vi "MouseDown.vi"(7 "Flip colors?":bool, 8 "error in":errorcluster, 10 "Coords":T5, 11 "Data in":T1={"Class"={"Ants"=refnum, "Layer"=refnum, "Templates"=refnum, "Icon"=refnum, "Glyph"=refnum, "Settings"=refnum, "Tools"=refnum, "History"=refnum}, "Ref"={"Add Layer"=refnum, "Remove Layer"=refnum, "Line Text"=[], "Body Text Spec"=refnum, "DNL_Font"=refnum, "glyph path str"=refnum, "templates path str"=refnum, "Arrow Up"=refnum, "Arrow Down"=refnum, "IE VI Ref"=refnum, "Glyphs tree"=refnum, "Templates tree"=refnum, "Layer Icon Text"=refnum, "Layer Template"=refnum, "Body Text"=refnum, "Search Templates"=refnum, "TextMarker"=refnum, "Tab Control"=refnum, "Search Glyphs"=refnum, "Line Color"=refnum, "DNL_Glyphs []"=refnum, "Fill Color"=refnum, "Tools"=refnum, "Icon"=refnum, "Preview"=refnum, "Ants"=refnum, "Terminals"=refnum, "menu reference"=refnum, "LayerNames"=[], "GlyphLoadAnimation"=refnum, "TemplateLoadAnimation"=refnum, "refreshGlyphs"=refnum, "refreshTemplates"=refnum}, "Support"={"AntsRect"={"left"=0, "top"=0, "right"=0, "bottom"=0}, "Mouse Move Coords"={"Horizontal"=0, "Vertical"=0}, "Mouse Down Coords"={"Horizontal"=0, "Vertical"=0}, "Temp Coord"={"Horizontal"=0, "Vertical"=0}, "Action"=enum."Default", "Edge Color"=4914962, "Fill Color"=16860, "Mouse Down?"=FALSE, "Draft Mode?"=FALSE, "Temp Icon"=bytes[3102], "CTRL Pressed"=FALSE, "Move Selection?"=FALSE, "AntsRect Orig"={"left"=0, "top"=0, "right"=0, "bottom"=0}, "Text"="", "TM Set?"=FALSE, "Mouse inside icon?"=FALSE, "Tool (old value)"=0, "Pencil Move Color"=0, "Swap Colors?"=FALSE, "Shift pressed?"=FALSE}}) -> (0 "error out":errorcluster, 3 "Data out":T1={"Class"={"Ants"=refnum, "Layer"=refnum, "Templates"=refnum, "Icon"=refnum, "Glyph"=refnum, "Settings"=refnum, "Tools"=refnum, "History"=refnum}, "Ref"={"Add Layer"=refnum, "Remove Layer"=refnum, "Line Text"=[], "Body Text Spec"=refnum, "DNL_Font"=refnum, "glyph path str"=refnum, "templates path str"=refnum, "Arrow Up"=refnum, "Arrow Down"=refnum, "IE VI Ref"=refnum, "Glyphs tree"=refnum, "Templates tree"=refnum, "Layer Icon Text"=refnum, "Layer Template"=refnum, "Body Text"=refnum, "Search Templates"=refnum, "TextMarker"=refnum, "Tab Control"=refnum, "Search Glyphs"=refnum, "Line Color"=refnum, "DNL_Glyphs []"=refnum, "Fill Color"=refnum, "Tools"=refnum, "Icon"=refnum, "Preview"=refnum, "Ants"=refnum, "Terminals"=refnum, "menu reference"=refnum, "LayerNames"=[], "GlyphLoadAnimation"=refnum, "TemplateLoadAnimation"=refnum, "refreshGlyphs"=refnum, "refreshTemplates"=refnum}, "Support"={"AntsRect"={"left"=0, "top"=0, "right"=0, "bottom"=0}, "Mouse Move Coords"={"Horizontal"=0, "Vertical"=0}, "Mouse Down Coords"={"Horizontal"=0, "Vertical"=0}, "Temp Coord"={"Horizontal"=0, "Vertical"=0}, "Action"=enum."Default", "Edge Color"=4914962, "Fill Color"=16860, "Mouse Down?"=FALSE, "Draft Mode?"=FALSE, "Temp Icon"=bytes[3102], "CTRL Pressed"=FALSE, "Move Selection?"=FALSE, "AntsRect Orig"={"left"=0, "top"=0, "right"=0, "bottom"=0}, "Text"="", "TM Set?"=FALSE, "Mouse inside icon?"=FALSE, "Tool (old value)"=0, "Pencil Move Color"=0, "Swap Colors?"=FALSE, "Shift pressed?"=FALSE}})   [LabVIEW 2020]
uses:
  Class/Ants/Ants.lvclass
  Class/FakedArray/FakedArray.lvclass
  vi.lib/LabVIEW Icon API/lv_icon/Classes/Icon/Icon.lvclass
  Class/Icon Library/Glyph.lvclass
  Class/Settings/Settings.lvclass
  Class/Tools/Tools Paint.lvclass
  History/History/History.lvclass
  Controls/SupportClass_Action.ctl
  History/History.lvlib
  <vilib>/Utility/miscctls.llb/LVPoint32TypeDef.ctl
  vi.lib/LabVIEW Icon API/lv_icon/Controls/IEColor.ctl
  Controls/Support Cluster.ctl
  lv_icon.lvlib
  Controls/References Cluster.ctl
  Controls/IE Classes.ctl
  Controls/Global Data.ctl
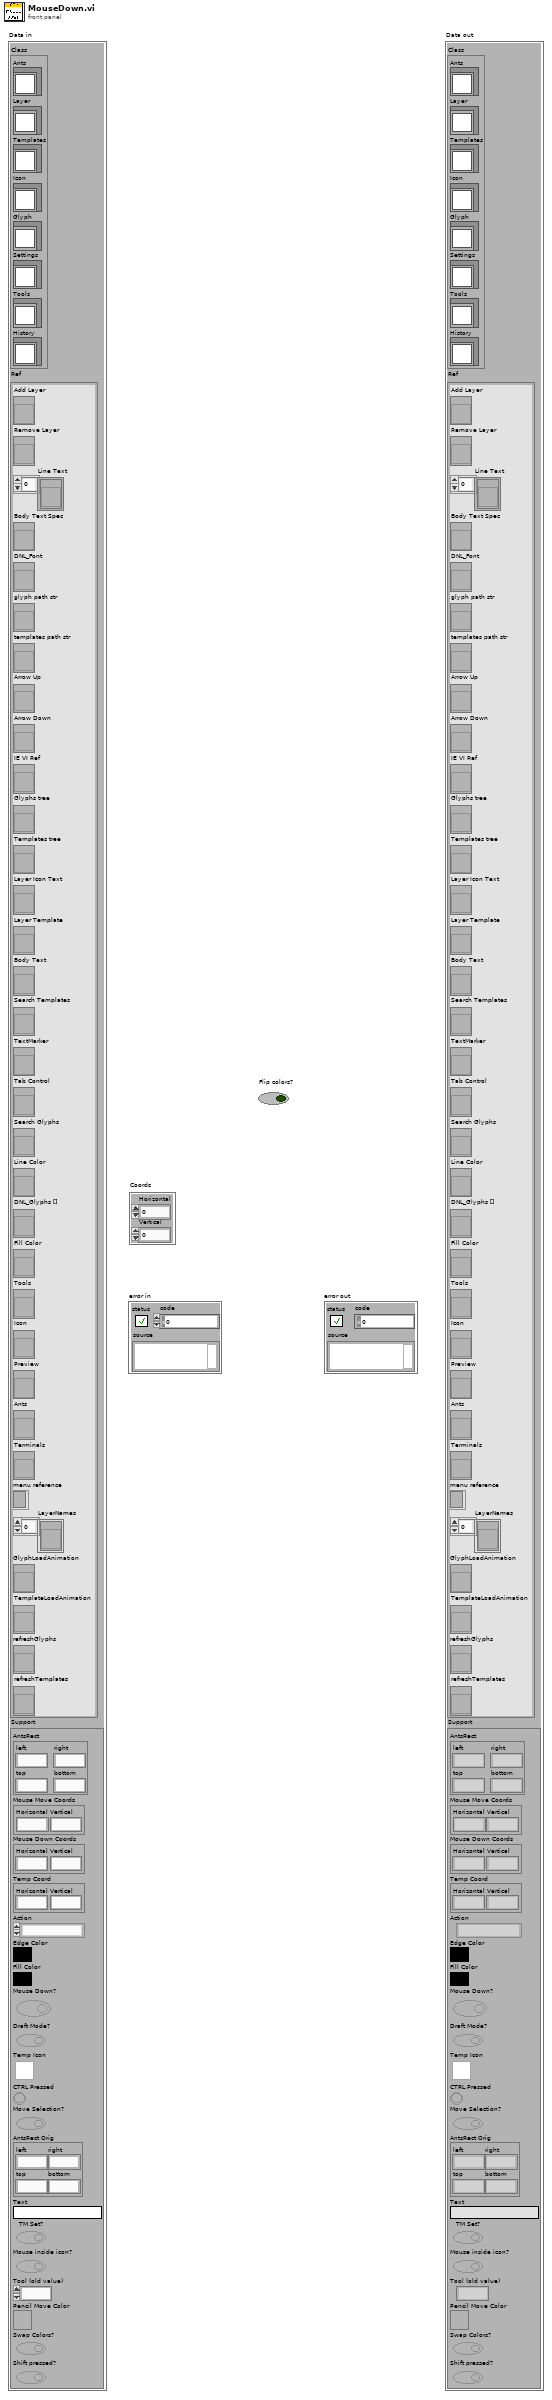
[diagram p1: front panel]
types:
  T1 = typedef "lv_icon.lvlib/Global Data.ctl" = cluster{"Class":T2, "Ref":T3, "Support":T4}
  T2 = typedef "lv_icon.lvlib/IE Classes.ctl" = cluster{"Ants":refnum<class "Ants.lvclass">, "Layer":refnum<class "FakedArray.lvclass">, "Templates":refnum<class "FakedArray.lvclass">, "Icon":refnum<class "Icon.lvclass">, "Glyph":refnum<class "Glyph.lvclass">, "Settings":refnum<class "Settings.lvclass">, "Tools":refnum<class "Tools Paint.lvclass">, "History":refnum<class "History.lvclass">}
  T3 = typedef "lv_icon.lvlib/References Cluster.ctl" = cluster{"Add Layer":refnum<vi>, "Remove Layer":refnum<vi>, "Line Text":refnum<vi>[], "Body Text Spec":refnum<vi>, "DNL_Font":refnum<vi>, "glyph path str":refnum<vi>, "templates path str":refnum<vi>, "Arrow Up":refnum<vi>, "Arrow Down":refnum<vi>, "IE VI Ref":refnum<vi>, "Glyphs tree":refnum<vi>, "Templates tree":refnum<vi>, "Layer Icon Text":refnum<vi>, "Layer Template":refnum<vi>, "Body Text":refnum<vi>, "Search Templates":refnum<vi>, "TextMarker":refnum<vi>, "Tab Control":refnum<vi>, "Search Glyphs":refnum<vi>, "Line Color":refnum<vi>, "DNL_Glyphs []":refnum<vi>, "Fill Color":refnum<vi>, "Tools":refnum<vi>, "Icon":refnum<vi>, "Preview":refnum<vi>, "Ants":refnum<vi>, "Terminals":refnum<vi>, "menu reference":refnum<k9>, "LayerNames":refnum<vi>[], "GlyphLoadAnimation":refnum<vi>, "TemplateLoadAnimation":refnum<vi>, "refreshGlyphs":refnum<vi>, "refreshTemplates":refnum<vi>}
  T4 = typedef "lv_icon.lvlib/Support Cluster.ctl" = cluster{"AntsRect":cluster{"left":i16, "top":i16, "right":i16, "bottom":i16}, "Mouse Move Coords":T5, "Mouse Down Coords":T5, "Temp Coord":T5, "Action":T6, "Edge Color":T7, "Fill Color":T7, "Mouse Down?":bool, "Draft Mode?":bool, "Temp Icon":picture, "CTRL Pressed":bool, "Move Selection?":bool, "AntsRect Orig":cluster{"left":i16, "top":i16, "right":i16, "bottom":i16}, "Text":string, "TM Set?":bool, "Mouse inside icon?":bool, "Tool (old value)":u32, "Pencil Move Color":u32, "Swap Colors?":bool, "Shift pressed?":bool}
  T5 = typedef "LVPoint32TypeDef.ctl" = cluster{"Horizontal":i32, "Vertical":i32}
  T6 = typedef "SupportClass_Action.ctl" = enum16{"Default", "Move Selection", "Glyph Library", "Tool"}
  T7 = typedef "IEColor.ctl" = u32
  T8 = cluster{"left":i16, "top":i16, "right":i16, "bottom":i16}
  T9 = typedef "Tools.ctl" = enum32{"Pencil", "Line", "Dropper", "Fill", "Rectangle", "Filled Rectangle", "Ellipse", "Filled Ellipse", "Eraser", "Text", "Select", "Move"}
  T10 = cluster{"Horizontal":i32, "Vertical":i32, "Vertical 2":i32, "Vertical 3":i32}
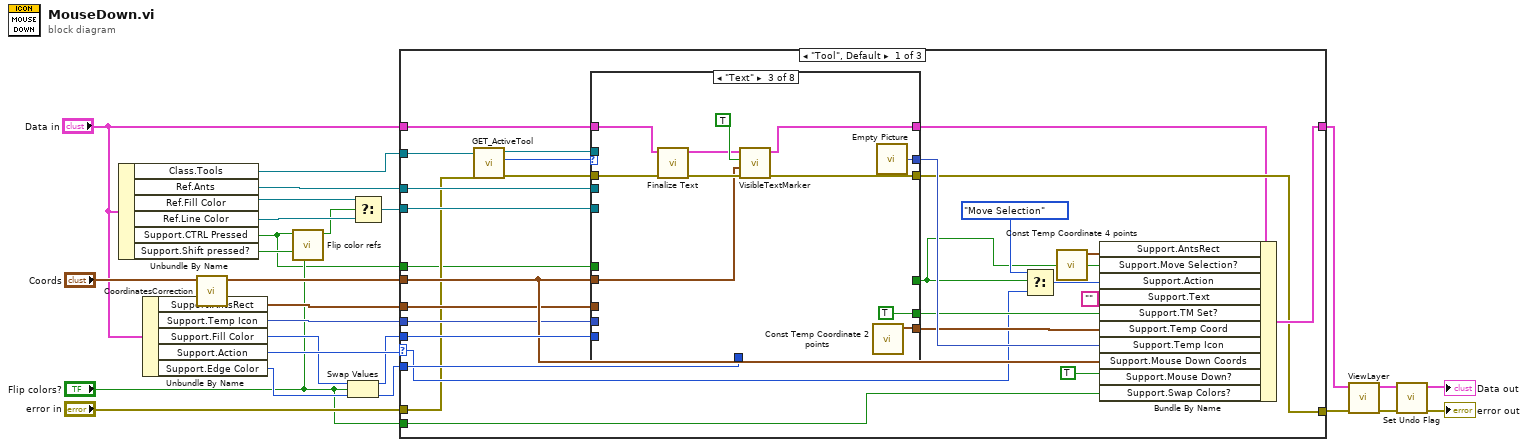
[diagram p0: block diagram]
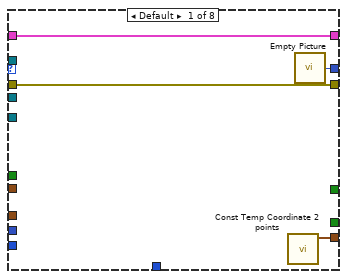
[diagram p2: hidden frame]
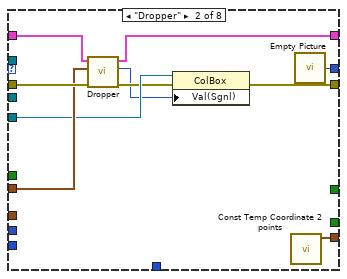
[diagram p3: hidden frame]
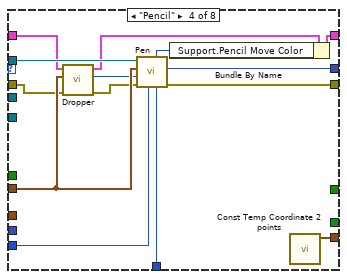
[diagram p4: hidden frame]
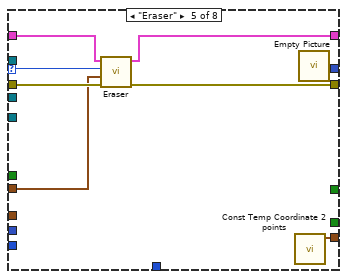
[diagram p5: hidden frame]
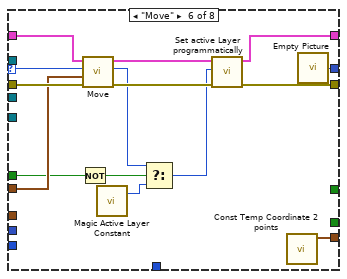
[diagram p6: hidden frame]
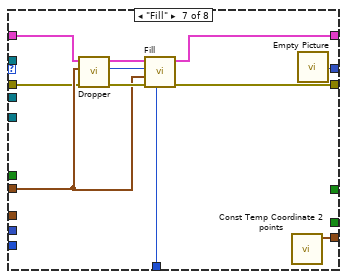
[diagram p7: hidden frame]
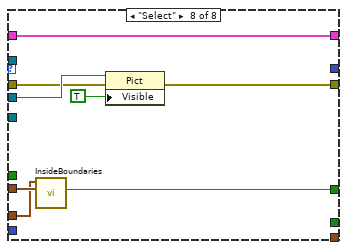
[diagram p8: hidden frame]
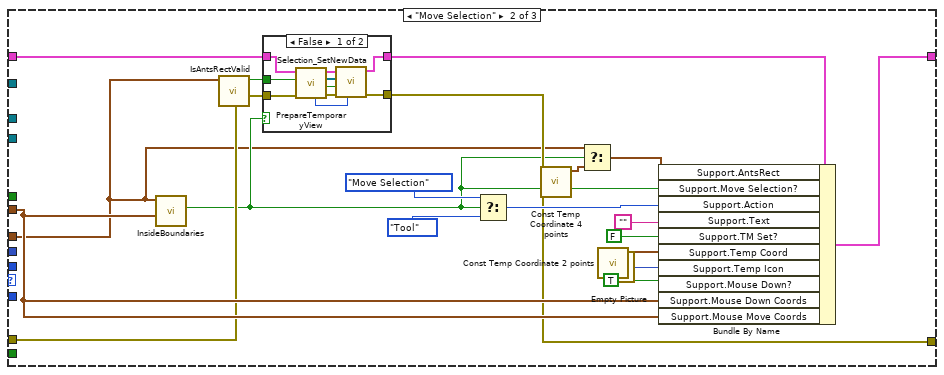
[diagram p9: hidden frame]
diagram:
  n1 = Unbundle By Name("Data in") -> ("Class.Tools"=w20:refnum<class "Tools Paint.lvclass">, "Ref.Ants"=w22:refnum<vi>, "Ref.Fill Color"=w9:refnum<vi>, "Ref.Line Color"=w8:refnum<vi>, "Support.CTRL Pressed"=w4:bool, "Support.Shift pressed?"=w5:bool)
  n2 = Unbundle By Name("Data in") -> ("Support.AntsRect"=w21:T8, "Support.Temp Icon"=w23:picture, "Support.Fill Color"=w12:T7, "Support.Action"=w25:T6, "Support.Edge Color"=w14:T7)
  n3 = call "CoordinatesCorrection.vi"("Coordinates In"="Coords") -> ("Corrected Out"=w26:T5)  [unwired: 10 out]
  n4 = call "Flip color refs.vi"("Flip colors?"="Flip colors?", "Shift pressed"=w5, "CTRL pressed"=w4) -> ("Flip?"=w6:bool)  [unwired: 8 out]
  n5 = Swap Values(12:w12, 13:"Flip colors?", 14:w14) -> (1:w11:T7, 3:w13:T7)
  n6 = Select(t=w9, s=w6, f=w8) -> (s? t:f=w10:refnum<vi>)
  n7 = case shown="\"Tool\", Default" w25 {
    selector: w25 -> [w39 _ _]
    tunnel: [w47 w142 w168] -> w17
    tunnel: w26 -> [w50 w145 _]
    tunnel: "error in" -> [w32 w143 w168]
    tunnel: [w48 w150 w167] -> w15
    tunnel: w11 -> [w51 _ _]
    tunnel: w13 -> [w46 _ _]
    tunnel: w23 -> [w43 _ _]
    tunnel: w22 -> [w42 _ _]
    tunnel: w21 -> [w41 w138 _]
    tunnel: w10 -> [w35 _ _]
    tunnel: w20 -> [w33 _ _]
    tunnel: "Data in" -> [w31 w141 w167]
    tunnel: "Flip colors?" -> [w30 _ _]
    tunnel: w4 -> [w28 _ _]
    frame "Tool", Default {
      n8 = call-dynamic "GET_ActiveTool.vi"("error in (no error)"=w32, "Tools Paint.lvclass in"=w33) -> ("error out"=w53:errorcluster, "Radio Buttons"=w54:T9, "Tools Paint.lvclass out"=w36:refnum<class "Tools Paint.lvclass">)  [unwired: 7 out]
      n9 = case shown="\"Text\"" w54 {
        selector: w54 -> [_ _ _ _ w97 w113 _ _]
        tunnel: w53 -> [w58 w67 w75 w88 w100 w115 w122 w129]
        tunnel: w50 -> [_ w65 w69 w89 w98 w114 w123 w132]
        tunnel: w51 -> [_ _ _ w80 _ _ _ _]
        tunnel: [w57 w68 w76 w93 w101 w116 w126 _] -> w49
        tunnel: [w58 w66 w78 w92 w99 w110 w125 w133] -> w47
        tunnel: w46 -> [_ _ _ w81 _ _ w117 _]
        tunnel: [w56 w64 w79 w91 w96 w112 w127 _] -> w45
        tunnel: [_ _ TRUE ("Mouse Down?") _ _ _ _ _] -> w44
        tunnel: w43 -> [_ _ _ _ _ _ _ _]
        tunnel: w42 -> [_ _ _ _ _ _ _ w135]
        tunnel: w41 -> [_ _ _ _ _ _ _ w131]
        tunnel: [_ _ _ _ _ _ _ w130] -> w34
        tunnel: w36 -> [_ _ _ w90 _ _ _ _]
        tunnel: w35 -> [_ w63 _ _ _ _ _ _]
        tunnel: w31 -> [w55 w62 w73 w85 w95 w109 w120 w128]
        tunnel: [w55 w61 w70 w83 w94 w107 w118 w128] -> w27
        tunnel: w28 -> [_ _ _ _ _ w106 _ _]
        frame Default {
          n10 = call "Const Temp Coordinate 2 points.vi"() -> ("Const Temp Coordinate"=w56:T5)  [unwired: 11 out]
          n11 = call "Empty Picture"() -> ("empty picture"=w57:picture)
        }
        frame "Dropper" {
          n12 = call "Dropper.vi"("error in (no error)"=w67, "point(x,y)"=w65, "Data in"=w62) -> ("error out"=w60:errorcluster, "Color"=w59:u32, "Data out"=w61:T1)  [unwired: 1 in, 5 out]
          n13 = property on="Property Node" class="ColBox"(reference=w63, error in=w60, "Val(Sgnl)"=w59) -> (error out=w66:errorcluster)  [unwired: 1 out]
          n14 = call "Const Temp Coordinate 2 points.vi"() -> ("Const Temp Coordinate"=w64:T5)  [unwired: 11 out]
          n15 = call "Empty Picture"() -> ("empty picture"=w68:picture)
        }
        frame "Text" {
          n16 = call "Finalize Text.vi"("error in (no error)"=w75, "Data in"=w73) -> ("error out"=w74:errorcluster, "Data out"=w71:T1)  [unwired: 8 out]
          n17 = call "VisibleTextMarker.vi"("error in (no error)"=w74, "Position"=w69, "Visible"=TRUE, "Data in"=w71) -> ("error out"=w78:errorcluster, "Data out"=w70:T1)  [unwired: 6 out]
          n18 = call "Const Temp Coordinate 2 points.vi"() -> ("Const Temp Coordinate"=w79:T5)  [unwired: 11 out]
          n19 = call "Empty Picture"() -> ("empty picture"=w76:picture)
        }
        frame "Pencil" {
          n20 = call "Dropper.vi"("error in (no error)"=w88, "point(x,y)"=w89, "Data in"=w85) -> ("error out"=w87:errorcluster, "Color"=w86:u32, "Data out"=w84:T1)  [unwired: 6 out]
          n21 = call-dynamic "Pen.vi"("Edge color"=w81, "Fill color"=w80, "error in (no error)"=w87, "Current color (T)"=w86, "point(x,y)"=w89, "Tools Paint in"=w90) -> ("error out"=w92:errorcluster, "new picture"=w93:picture, "Current line color"=w82:u32)  [unwired: 3 out]
          n22 = Bundle By Name(cluster=w84, "Support.Pencil Move Color"=w82) -> (w83:T1)
          n23 = call "Const Temp Coordinate 2 points.vi"() -> ("Const Temp Coordinate"=w91:T5)  [unwired: 11 out]
        }
        frame "Eraser" {
          n24 = call "Eraser.vi"("error in (no error)"=w100, "point(x,y)"=w98, "Radio Buttons"=w97, "Data in"=w95) -> ("error out"=w99:errorcluster, "Data out"=w94:T1)  [unwired: 1 in, 5 out]
          n25 = call "Const Temp Coordinate 2 points.vi"() -> ("Const Temp Coordinate"=w96:T5)  [unwired: 11 out]
          n26 = call "Empty Picture"() -> ("empty picture"=w101:picture)
        }
        frame "Move" {
          n27 = Not(x=w106) -> (.not. x?=w105:bool)
          n28 = call "Move.vi"("error in (no error)"=w115, "point(x,y)"=w114, "Tools"=w113, "Data in"=w109) -> ("error out"=w111:errorcluster, "Active Layer"=w104:i32, "Data out"=w108:T1)  [unwired: 1 in, 4 out]
          n29 = call "Magic Active Layer Constant.vi"() -> ("Magic Constant"=w103:i32)  [unwired: 19 out]
          n30 = Select(t=w104, s=w105, f=w103) -> (s? t:f=w102:i32)
          n31 = call "Set active Layer programmatically.vi"("error in"=w111, "Active Layer"=w102, "Data in"=w108) -> ("error out"=w110:errorcluster, "Data out"=w107:T1)  [unwired: 1 in, 6 out]
          n32 = call "Const Temp Coordinate 2 points.vi"() -> ("Const Temp Coordinate"=w112:T5)  [unwired: 11 out]
          n33 = call "Empty Picture"() -> ("empty picture"=w116:picture)
        }
        frame "Fill" {
          n34 = call "Dropper.vi"("error in (no error)"=w122, "point(x,y)"=w123, "Data in"=w120) -> ("error out"=w124:errorcluster, "Color"=w121:u32, "Data out"=w119:T1)  [unwired: 6 out]
          n35 = call "Fill.vi"("Color"=w117, "error in (no error)"=w124, "point(x,y)"=w123, "Ref Color"=w121, "Data in"=w119) -> ("error out"=w125:errorcluster, "Data out"=w118:T1)  [unwired: 1 in, 4 out]
          n36 = call "Const Temp Coordinate 2 points.vi"() -> ("Const Temp Coordinate"=w127:T5)  [unwired: 11 out]
          n37 = call "Empty Picture"() -> ("empty picture"=w126:picture)
        }
        frame "Select" {
          n38 = call "InsideBoundaries.vi"("Mouse Move Coords"=w132, "AntsRect"=w131) -> ("Inside?"=w130:bool)  [unwired: 9 out]
          n39 = property class="Pict"(reference=w135, error in=w129, "Visible"=TRUE) -> (error out=w133:errorcluster)  [unwired: 1 out]
        }
      }
      n40 = Select(t=SupportClass_Action."Move Selection", s=w34, f=w39) -> (s? t:f=w37:T6)
      n41 = call "Const Temp Coordinate 4 points.vi"() -> ("Const Temp Coordinate"=w29:T10)  [unwired: 11 out]
      n42 = Bundle By Name(cluster=w27, "Support.AntsRect"=w29, "Support.Move Selection?"=w34, "Support.Action"=w37, "Support.Text"="", "Support.TM Set?"=w44, "Support.Temp Coord"=w45, "Support.Temp Icon"=w49, "Support.Mouse Down Coords"=w50, "Support.Mouse Down?"=TRUE ("Mouse Down?"), "Support.Swap Colors?"=w30) -> (w48:T1)
    }
    frame "Move Selection" {
      n43 = call "InsideBoundaries.vi"("Mouse Move Coords"=w145, "AntsRect"=w138) -> ("Inside?"=w139:bool)  [unwired: 9 out]
      n44 = call "IsAntsRectValid.vi"("AntsRect"=w138) -> ("Valid?"=w144:bool)  [unwired: 10 out]
      n45 = case shown="False" w139 {
        tunnel: w144 -> [w161 _]
        tunnel: w143 -> [w160 w166]
        tunnel: [w159 w166] -> w142
        tunnel: w141 -> [w157 w165]
        tunnel: [w155 w165] -> w140
        frame False {
          n46 = call "PrepareTemporaryView.vi"("error in (no error)"=w160, "Valid Selection?"=w161, "Data in"=w157) -> ("error out"=w158:errorcluster, "Highlighted?"=w163:bool, "All Layers out"=w164:refnum<class "Layer.lvclass">[], "Data out"=w156:T1, "#Active Layer"=w162:i32)  [unwired: 2 in, 2 out]
          n47 = call "Selection_SetNewData.vi"("#Active Layer"=w162, "error in"=w158, "Highlighted?"=w163, "All Layers In"=w164, "Data in"=w156) -> ("error out"=w159:errorcluster, "Data out"=w155:T1)  [unwired: 1 in, 3 out]
        }
        frame True {
        }
      }
      n48 = Select(t=SupportClass_Action."Move Selection", s=w139, f=SupportClass_Action."Tool") -> (s? t:f=w149:T6)
      n49 = call "Const Temp Coordinate 4 points.vi"() -> ("Const Temp Coordinate"=w137:T10)  [unwired: 11 out]
      n50 = Select(t=w138, s=w139, f=w137) -> (s? t:f=w136:T10)
      n51 = call "Const Temp Coordinate 2 points.vi"() -> ("Const Temp Coordinate"=w148:T5)  [unwired: 11 out]
      n52 = call "Empty Picture"() -> ("empty picture"=w147:picture)
      n53 = Bundle By Name(cluster=w140, "Support.AntsRect"=w136, "Support.Move Selection?"=w139, "Support.Action"=w149, "Support.Text"="", "Support.TM Set?"=FALSE ("TM Set?"), "Support.Temp Coord"=w148, "Support.Temp Icon"=w147, "Support.Mouse Down?"=TRUE ("Mouse Down?"), "Support.Mouse Down Coords"=w145, "Support.Mouse Move Coords"=w145) -> (w150:T1)
    }
    frame "Glyph Library" {
    }
  }
  n54 = call "ViewLayer.vi"("error in (no error)"=w17, "Data in"=w15) -> ("error out"=w16:errorcluster, "Data out"=w2:T1)  [unwired: 2 in, 6 out]
  n55 = call "Set Undo Flag.vi"("error in"=w16, "Data in"=w2) -> ("error out"=→"error out":errorcluster, "Data out"=→"Data out":T1)  [unwired: 8 in]
